vi "Draw Stage Representation.vi"(9 "Well radius":i16=15, 10 "Well Spacing":i16=50, 11 "Area Size":cluster{"width":i16, "height":i16}) -> (2 "Well Spacing out":i16=50, 3 "new picture":picture)   [LabVIEW 2013, in "Microscope.lvclass"]
uses:
  Microscope.lvclass
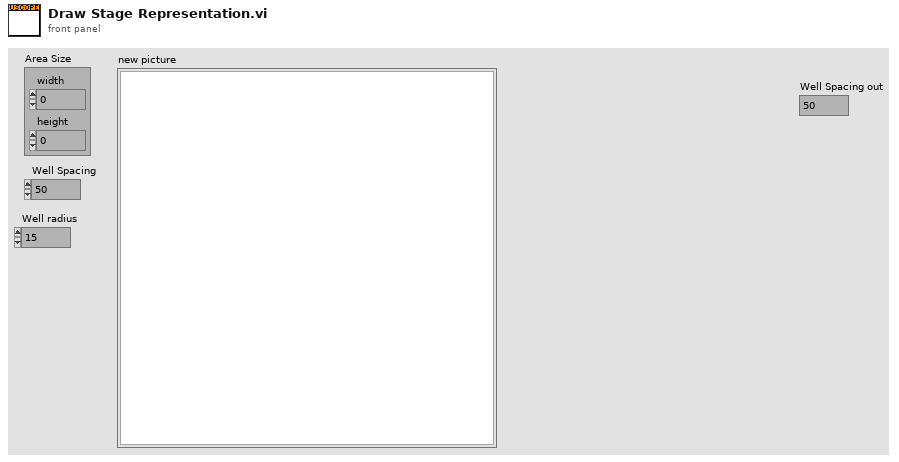
[diagram p1: front panel]
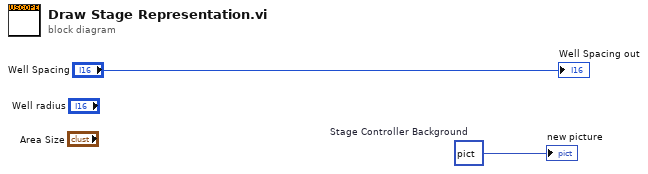
[diagram p0: block diagram]
diagram:
  w1 = picture bytes[419658]  # Stage Controller Background
  "new picture" <- w1
  "Well Spacing out" <- "Well Spacing"
